vi "ParseSlaveRY.vi"(0 "RY":bool[][](array[boolean])) -> (1 "PLC状态":T1, 2 "检测步骤":T2)   [LabVIEW 2018]
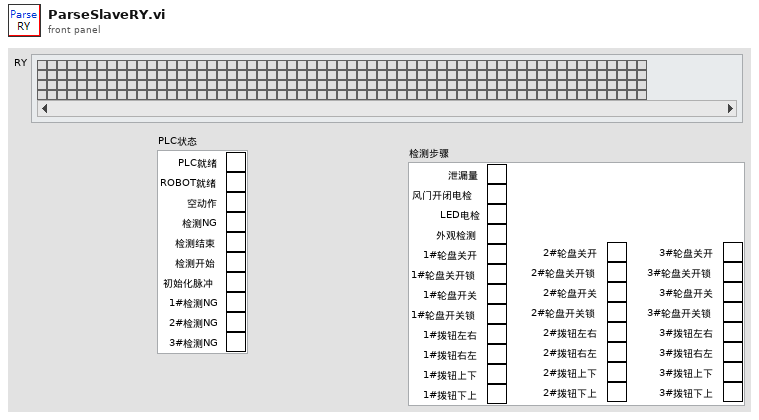
[diagram p1: front panel]
types:
  T1 = cluster{"PLC就绪":bool, "ROBOT就绪":bool, "空动作":bool, "检测NG":bool, "检测结束":bool, "检测开始":bool, "初始化脉冲":bool, "1#检测NG":bool, "2#检测NG":bool, "3#检测NG":bool}
  T2 = cluster{"泄漏量":bool, "风门开闭电检":bool, "LED电检":bool, "外观检测":bool, "1#轮盘关开":bool, "1#轮盘关开锁":bool, "1#轮盘开关":bool, "1#轮盘开关锁":bool, "1#拨钮左右":bool, "1#拨钮右左":bool, "1#拨钮上下":bool, "1#拨钮下上":bool, "2#轮盘关开":bool, "2#轮盘关开锁":bool, "2#轮盘开关":bool, "2#轮盘开关锁":bool, "2#拨钮左右":bool, "2#拨钮右左":bool, "2#拨钮上下":bool, "2#拨钮下上":bool, "3#轮盘关开":bool, "3#轮盘关开锁":bool, "3#轮盘开关":bool, "3#轮盘开关锁":bool, "3#拨钮左右":bool, "3#拨钮右左":bool, "3#拨钮上下":bool, "3#拨钮下上":bool}
  T3 = cluster{"1#泄漏量":bool, "1#风门闭电压":bool, "1#风门开电压":bool, "1#LED电压":bool, "1#LED电流":bool, "外观结果":bool, "2#泄漏量":bool, "2#风门闭电压":bool, "2#风门开电压":bool, "2#LED电压":bool, "2#LED电流":bool, "3#泄漏量":bool, "3#风门闭电压":bool, "3#风门开电压":bool, "3#LED电压":bool, "3#LED电流":bool}
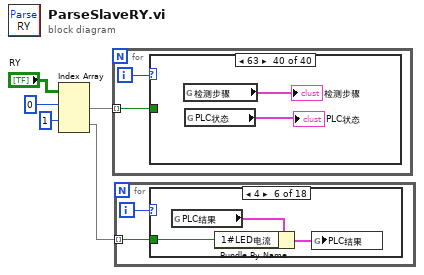
[diagram p0: block diagram]
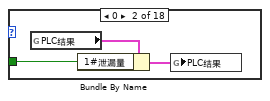
[diagram p3: hidden frame]
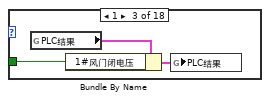
[diagram p4: hidden frame]
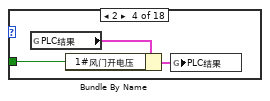
[diagram p5: hidden frame]
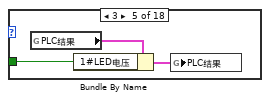
[diagram p6: hidden frame]
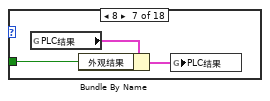
[diagram p7: hidden frame]
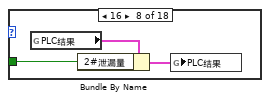
[diagram p8: hidden frame]
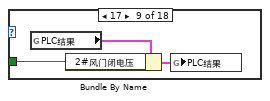
[diagram p9: hidden frame]
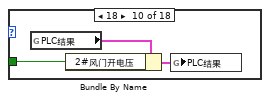
[diagram p10: hidden frame]
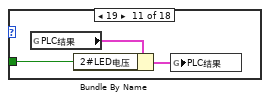
[diagram p11: hidden frame]
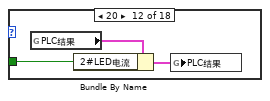
[diagram p12: hidden frame]
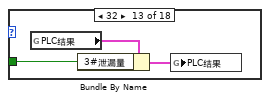
[diagram p13: hidden frame]
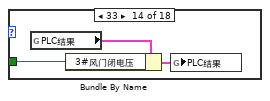
[diagram p14: hidden frame]
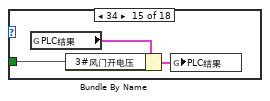
[diagram p15: hidden frame]
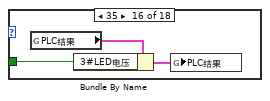
[diagram p16: hidden frame]
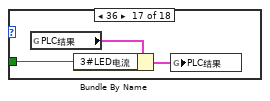
[diagram p17: hidden frame]
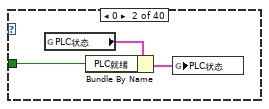
[diagram p20: hidden frame]
diagram:
  n1 = Index Array(array="RY", index (row) #1=0 ("索引 (行)"), index (row) #2=1 ("索引 (行)")) -> (element #1=w3:bool[], element #2=w1:bool[])  [unwired: 2 in]
  n2 = for {
    tunnel: w3 -> [w6] mode=indexing
    i -> [w7]
    n3 = case shown="63" w7 {
      tunnel: w6 -> [_ w9 w12 w15 w18 w21 w24 w27 w30 w33 w36 w38 w41 w44 w48 w51 w54 w57 w60 w63 w66 w69 w72 w75 w78 w81 w84 w87 w90 w93 w96 w99 w102 w105 w108 w111 w114 w117 w120 _]
      frame -1, Default {
      }
      frame 0 {
        n4 = global read "全局 1.vi" "PLC状态"() -> (w10:T1)
        n5 = Bundle By Name(cluster=w10, "PLC就绪"=w9) -> (w8:T1)
        n6 = global write "全局 1.vi" "PLC状态"(w8) -> ()
      }
      frame 1 {
        n7 = global read "全局 1.vi" "PLC状态"() -> (w13:T1)
        n8 = Bundle By Name(cluster=w13, "ROBOT就绪"=w12) -> (w11:T1)
        n9 = global write "全局 1.vi" "PLC状态"(w11) -> ()
      }
      frame 2 {
        n10 = global read "全局 1.vi" "PLC状态"() -> (w16:T1)
        n11 = Bundle By Name(cluster=w16, "空动作"=w15) -> (w14:T1)
        n12 = global write "全局 1.vi" "PLC状态"(w14) -> ()
      }
      frame 3 {
        n13 = global read "全局 1.vi" "PLC状态"() -> (w19:T1)
        n14 = Bundle By Name(cluster=w19, "检测NG"=w18) -> (w17:T1)
        n15 = global write "全局 1.vi" "PLC状态"(w17) -> ()
      }
      frame 4 {
        n16 = global read "全局 1.vi" "PLC状态"() -> (w22:T1)
        n17 = Bundle By Name(cluster=w22, "检测结束"=w21) -> (w20:T1)
        n18 = global write "全局 1.vi" "PLC状态"(w20) -> ()
      }
      frame 5 {
        n19 = global read "全局 1.vi" "PLC状态"() -> (w25:T1)
        n20 = Bundle By Name(cluster=w25, "检测开始"=w24) -> (w23:T1)
        n21 = global write "全局 1.vi" "PLC状态"(w23) -> ()
      }
      frame 6 {
        n22 = global read "全局 1.vi" "PLC状态"() -> (w28:T1)
        n23 = Bundle By Name(cluster=w28, "初始化脉冲"=w27) -> (w26:T1)
        n24 = global write "全局 1.vi" "PLC状态"(w26) -> ()
      }
      frame 8 {
        n25 = global read "全局 1.vi" "PLC状态"() -> (w31:T1)
        n26 = Bundle By Name(cluster=w31, "1#检测NG"=w30) -> (w29:T1)
        n27 = global write "全局 1.vi" "PLC状态"(w29) -> ()
      }
      frame 9 {
        n28 = global read "全局 1.vi" "PLC状态"() -> (w34:T1)
        n29 = Bundle By Name(cluster=w34, "2#检测NG"=w33) -> (w32:T1)
        n30 = global write "全局 1.vi" "PLC状态"(w32) -> ()
      }
      frame 10 {
        n31 = global read "全局 1.vi" "PLC状态"() -> (w37:T1)
        n32 = Bundle By Name(cluster=w37, "3#检测NG"=w36) -> (w35:T1)
        n33 = global write "全局 1.vi" "PLC状态"(w35) -> ()
      }
      frame 16 {
        n34 = global read "全局 1.vi" "检测步骤"() -> (w40:T2)
        n35 = Bundle By Name(cluster=w40, "泄漏量"=w38) -> (w39:T2)
        n36 = global write "全局 1.vi" "检测步骤"(w39) -> ()
      }
      frame 17 {
        n37 = global read "全局 1.vi" "检测步骤"() -> (w43:T2)
        n38 = Bundle By Name(cluster=w43, "风门开闭电检"=w41) -> (w42:T2)
        n39 = global write "全局 1.vi" "检测步骤"(w42) -> ()
      }
      frame 18 {
        n40 = global read "全局 1.vi" "检测步骤"() -> (w46:T2)
        n41 = Bundle By Name(cluster=w46, "LED电检"=w44) -> (w45:T2)
        n42 = global write "全局 1.vi" "检测步骤"(w45) -> ()
      }
      frame 25 {
        n43 = global read "全局 1.vi" "检测步骤"() -> (w49:T2)
        n44 = Bundle By Name(cluster=w49, "外观检测"=w48) -> (w47:T2)
        n45 = global write "全局 1.vi" "检测步骤"(w47) -> ()
      }
      frame 32 {
        n46 = global read "全局 1.vi" "检测步骤"() -> (w52:T2)
        n47 = Bundle By Name(cluster=w52, "1#轮盘关开"=w51) -> (w50:T2)
        n48 = global write "全局 1.vi" "检测步骤"(w50) -> ()
      }
      frame 33 {
        n49 = global read "全局 1.vi" "检测步骤"() -> (w55:T2)
        n50 = Bundle By Name(cluster=w55, "1#轮盘关开锁"=w54) -> (w53:T2)
        n51 = global write "全局 1.vi" "检测步骤"(w53) -> ()
      }
      frame 34 {
        n52 = global read "全局 1.vi" "检测步骤"() -> (w58:T2)
        n53 = Bundle By Name(cluster=w58, "1#轮盘开关"=w57) -> (w56:T2)
        n54 = global write "全局 1.vi" "检测步骤"(w56) -> ()
      }
      frame 35 {
        n55 = global read "全局 1.vi" "检测步骤"() -> (w61:T2)
        n56 = Bundle By Name(cluster=w61, "1#轮盘开关锁"=w60) -> (w59:T2)
        n57 = global write "全局 1.vi" "检测步骤"(w59) -> ()
      }
      frame 36 {
        n58 = global read "全局 1.vi" "检测步骤"() -> (w64:T2)
        n59 = Bundle By Name(cluster=w64, "1#拨钮左右"=w63) -> (w62:T2)
        n60 = global write "全局 1.vi" "检测步骤"(w62) -> ()
      }
      frame 37 {
        n61 = global read "全局 1.vi" "检测步骤"() -> (w67:T2)
        n62 = Bundle By Name(cluster=w67, "1#拨钮右左"=w66) -> (w65:T2)
        n63 = global write "全局 1.vi" "检测步骤"(w65) -> ()
      }
      frame 38 {
        n64 = global read "全局 1.vi" "检测步骤"() -> (w70:T2)
        n65 = Bundle By Name(cluster=w70, "1#拨钮上下"=w69) -> (w68:T2)
        n66 = global write "全局 1.vi" "检测步骤"(w68) -> ()
      }
      frame 39 {
        n67 = global read "全局 1.vi" "检测步骤"() -> (w73:T2)
        n68 = Bundle By Name(cluster=w73, "1#拨钮下上"=w72) -> (w71:T2)
        n69 = global write "全局 1.vi" "检测步骤"(w71) -> ()
      }
      frame 40 {
        n70 = global read "全局 1.vi" "检测步骤"() -> (w76:T2)
        n71 = Bundle By Name(cluster=w76, "2#轮盘关开"=w75) -> (w74:T2)
        n72 = global write "全局 1.vi" "检测步骤"(w74) -> ()
      }
      frame 41 {
        n73 = global read "全局 1.vi" "检测步骤"() -> (w79:T2)
        n74 = Bundle By Name(cluster=w79, "2#轮盘关开锁"=w78) -> (w77:T2)
        n75 = global write "全局 1.vi" "检测步骤"(w77) -> ()
      }
      frame 42 {
        n76 = global read "全局 1.vi" "检测步骤"() -> (w82:T2)
        n77 = Bundle By Name(cluster=w82, "2#轮盘开关"=w81) -> (w80:T2)
        n78 = global write "全局 1.vi" "检测步骤"(w80) -> ()
      }
      frame 43 {
        n79 = global read "全局 1.vi" "检测步骤"() -> (w85:T2)
        n80 = Bundle By Name(cluster=w85, "2#轮盘开关锁"=w84) -> (w83:T2)
        n81 = global write "全局 1.vi" "检测步骤"(w83) -> ()
      }
      frame 44 {
        n82 = global read "全局 1.vi" "检测步骤"() -> (w88:T2)
        n83 = Bundle By Name(cluster=w88, "2#拨钮左右"=w87) -> (w86:T2)
        n84 = global write "全局 1.vi" "检测步骤"(w86) -> ()
      }
      frame 45 {
        n85 = global read "全局 1.vi" "检测步骤"() -> (w91:T2)
        n86 = Bundle By Name(cluster=w91, "2#拨钮右左"=w90) -> (w89:T2)
        n87 = global write "全局 1.vi" "检测步骤"(w89) -> ()
      }
      frame 46 {
        n88 = global read "全局 1.vi" "检测步骤"() -> (w94:T2)
        n89 = Bundle By Name(cluster=w94, "2#拨钮上下"=w93) -> (w92:T2)
        n90 = global write "全局 1.vi" "检测步骤"(w92) -> ()
      }
      frame 47 {
        n91 = global read "全局 1.vi" "检测步骤"() -> (w97:T2)
        n92 = Bundle By Name(cluster=w97, "2#拨钮下上"=w96) -> (w95:T2)
        n93 = global write "全局 1.vi" "检测步骤"(w95) -> ()
      }
      frame 48 {
        n94 = global read "全局 1.vi" "检测步骤"() -> (w100:T2)
        n95 = Bundle By Name(cluster=w100, "3#轮盘关开"=w99) -> (w98:T2)
        n96 = global write "全局 1.vi" "检测步骤"(w98) -> ()
      }
      frame 49 {
        n97 = global read "全局 1.vi" "检测步骤"() -> (w103:T2)
        n98 = Bundle By Name(cluster=w103, "3#轮盘关开锁"=w102) -> (w101:T2)
        n99 = global write "全局 1.vi" "检测步骤"(w101) -> ()
      }
      frame 50 {
        n100 = global read "全局 1.vi" "检测步骤"() -> (w106:T2)
        n101 = Bundle By Name(cluster=w106, "3#轮盘开关"=w105) -> (w104:T2)
        n102 = global write "全局 1.vi" "检测步骤"(w104) -> ()
      }
      frame 51 {
        n103 = global read "全局 1.vi" "检测步骤"() -> (w109:T2)
        n104 = Bundle By Name(cluster=w109, "3#轮盘开关锁"=w108) -> (w107:T2)
        n105 = global write "全局 1.vi" "检测步骤"(w107) -> ()
      }
      frame 52 {
        n106 = global read "全局 1.vi" "检测步骤"() -> (w112:T2)
        n107 = Bundle By Name(cluster=w112, "3#拨钮左右"=w111) -> (w110:T2)
        n108 = global write "全局 1.vi" "检测步骤"(w110) -> ()
      }
      frame 53 {
        n109 = global read "全局 1.vi" "检测步骤"() -> (w115:T2)
        n110 = Bundle By Name(cluster=w115, "3#拨钮右左"=w114) -> (w113:T2)
        n111 = global write "全局 1.vi" "检测步骤"(w113) -> ()
      }
      frame 54 {
        n112 = global read "全局 1.vi" "检测步骤"() -> (w118:T2)
        n113 = Bundle By Name(cluster=w118, "3#拨钮上下"=w117) -> (w116:T2)
        n114 = global write "全局 1.vi" "检测步骤"(w116) -> ()
      }
      frame 55 {
        n115 = global read "全局 1.vi" "检测步骤"() -> (w121:T2)
        n116 = Bundle By Name(cluster=w121, "3#拨钮下上"=w120) -> (w119:T2)
        n117 = global write "全局 1.vi" "检测步骤"(w119) -> ()
      }
      frame 63 {
        n118 = global read "全局 1.vi" "检测步骤"() -> (→"检测步骤":T2)
        n119 = global read "全局 1.vi" "PLC状态"() -> (→"PLC状态":T1)
      }
    }
  }
  n120 = for {
    tunnel: w1 -> [w124] mode=indexing
    i -> [w125]
    n121 = case shown="4" w125 {
      tunnel: w124 -> [_ w126 w129 w132 w135 w138 w141 w144 w147 w150 w153 w156 w159 w162 w165 w168 w171 _]
      frame -1, Default {
      }
      frame 0 {
        n122 = global read "全局 1.vi" "PLC结果"() -> (w128:T3)
        n123 = Bundle By Name(cluster=w128, "1#泄漏量"=w126) -> (w127:T3)
        n124 = global write "全局 1.vi" "PLC结果"(w127) -> ()
      }
      frame 1 {
        n125 = global read "全局 1.vi" "PLC结果"() -> (w131:T3)
        n126 = Bundle By Name(cluster=w131, "1#风门闭电压"=w129) -> (w130:T3)
        n127 = global write "全局 1.vi" "PLC结果"(w130) -> ()
      }
      frame 2 {
        n128 = global read "全局 1.vi" "PLC结果"() -> (w134:T3)
        n129 = Bundle By Name(cluster=w134, "1#风门开电压"=w132) -> (w133:T3)
        n130 = global write "全局 1.vi" "PLC结果"(w133) -> ()
      }
      frame 3 {
        n131 = global read "全局 1.vi" "PLC结果"() -> (w137:T3)
        n132 = Bundle By Name(cluster=w137, "1#LED电压"=w135) -> (w136:T3)
        n133 = global write "全局 1.vi" "PLC结果"(w136) -> ()
      }
      frame 4 {
        n134 = global read "全局 1.vi" "PLC结果"() -> (w140:T3)
        n135 = Bundle By Name(cluster=w140, "1#LED电流"=w138) -> (w139:T3)
        n136 = global write "全局 1.vi" "PLC结果"(w139) -> ()
      }
      frame 8 {
        n137 = global read "全局 1.vi" "PLC结果"() -> (w143:T3)
        n138 = Bundle By Name(cluster=w143, "外观结果"=w141) -> (w142:T3)
        n139 = global write "全局 1.vi" "PLC结果"(w142) -> ()
      }
      frame 16 {
        n140 = global read "全局 1.vi" "PLC结果"() -> (w146:T3)
        n141 = Bundle By Name(cluster=w146, "2#泄漏量"=w144) -> (w145:T3)
        n142 = global write "全局 1.vi" "PLC结果"(w145) -> ()
      }
      frame 17 {
        n143 = global read "全局 1.vi" "PLC结果"() -> (w149:T3)
        n144 = Bundle By Name(cluster=w149, "2#风门闭电压"=w147) -> (w148:T3)
        n145 = global write "全局 1.vi" "PLC结果"(w148) -> ()
      }
      frame 18 {
        n146 = global read "全局 1.vi" "PLC结果"() -> (w152:T3)
        n147 = Bundle By Name(cluster=w152, "2#风门开电压"=w150) -> (w151:T3)
        n148 = global write "全局 1.vi" "PLC结果"(w151) -> ()
      }
      frame 19 {
        n149 = global read "全局 1.vi" "PLC结果"() -> (w155:T3)
        n150 = Bundle By Name(cluster=w155, "2#LED电压"=w153) -> (w154:T3)
        n151 = global write "全局 1.vi" "PLC结果"(w154) -> ()
      }
      frame 20 {
        n152 = global read "全局 1.vi" "PLC结果"() -> (w158:T3)
        n153 = Bundle By Name(cluster=w158, "2#LED电流"=w156) -> (w157:T3)
        n154 = global write "全局 1.vi" "PLC结果"(w157) -> ()
      }
      frame 32 {
        n155 = global read "全局 1.vi" "PLC结果"() -> (w161:T3)
        n156 = Bundle By Name(cluster=w161, "3#泄漏量"=w159) -> (w160:T3)
        n157 = global write "全局 1.vi" "PLC结果"(w160) -> ()
      }
      frame 33 {
        n158 = global read "全局 1.vi" "PLC结果"() -> (w164:T3)
        n159 = Bundle By Name(cluster=w164, "3#风门闭电压"=w162) -> (w163:T3)
        n160 = global write "全局 1.vi" "PLC结果"(w163) -> ()
      }
      frame 34 {
        n161 = global read "全局 1.vi" "PLC结果"() -> (w167:T3)
        n162 = Bundle By Name(cluster=w167, "3#风门开电压"=w165) -> (w166:T3)
        n163 = global write "全局 1.vi" "PLC结果"(w166) -> ()
      }
      frame 35 {
        n164 = global read "全局 1.vi" "PLC结果"() -> (w170:T3)
        n165 = Bundle By Name(cluster=w170, "3#LED电压"=w168) -> (w169:T3)
        n166 = global write "全局 1.vi" "PLC结果"(w169) -> ()
      }
      frame 36 {
        n167 = global read "全局 1.vi" "PLC结果"() -> (w173:T3)
        n168 = Bundle By Name(cluster=w173, "3#LED电流"=w171) -> (w172:T3)
        n169 = global write "全局 1.vi" "PLC结果"(w172) -> ()
      }
      frame 63 {
      }
    }
  }
